vi "Build Response.vi"(6 "Target ID":u8, 8 "Data 3":u16, 9 "Data 2":u16, 10 "Data 1":u16, 11 "Response":u8) -> (3 "Response Value":u64)   [LabVIEW 2020, in "BCI-1553 RT Interface.lvlib"]
uses:
  BCI-1553 RT Interface.lvlib
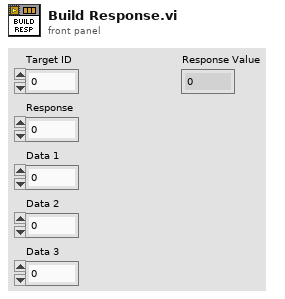
[diagram p1: front panel]
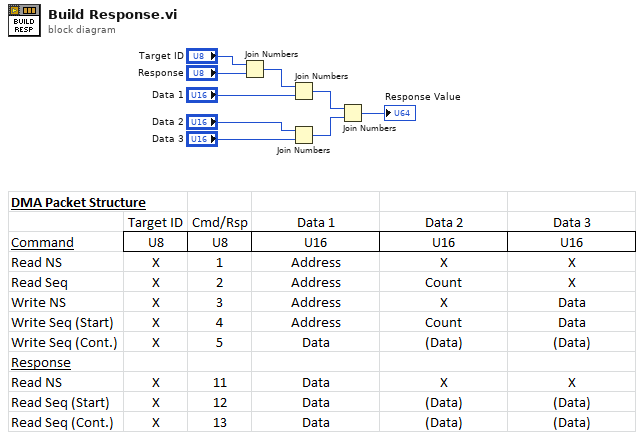
[diagram p0: block diagram]
diagram:
  n1 = Join Numbers(hi="Target ID", lo="Response") -> ((hi.lo)=w9:u16)
  n2 = Join Numbers(hi=w9, lo="Data 1") -> ((hi.lo)=w8:u32)
  n3 = Join Numbers(hi="Data 2", lo="Data 3") -> ((hi.lo)=w7:u32)
  n4 = Join Numbers(hi=w8, lo=w7) -> ((hi.lo)=→"Response Value":u64)
